vi "GetClusterElementByName(DBL).vi"(10 "ElementName":string[](array[string]), 11 "Cluster":variant) -> (2 "Found":bool, 3 "ValueOut":dbl)   [LabVIEW 2020, in "GetClusterElementByName.lvlib"]
uses:
  GetClusterElementByName.lvlib
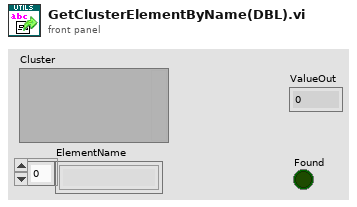
[diagram p1: front panel]
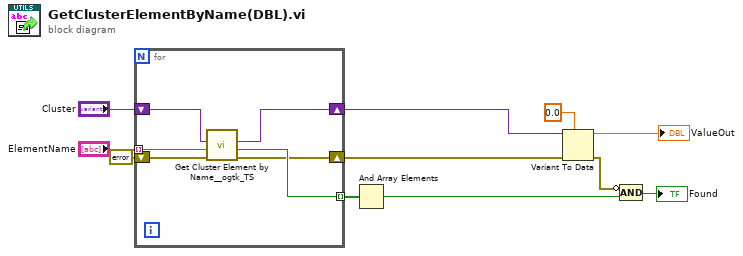
[diagram p0: block diagram]
diagram:
  n1 = for {
    tunnel: "ElementName" -> [w17] mode=indexing
    shift-right: [w16] -> w8
    shift-left: "Cluster" -> [w15]
    tunnel: [w14] -> w9 mode=indexing
    shift-right: [w13] -> w6
    shift-left: errorcluster {"status"=FALSE, "code"=0, "source"=""} ("error out") -> [w12]
    n2 = call "Get Cluster Element by Name__ogtk_TS.vi"("error in (no error)"=w12, "Element Name"=w17, "Cluster"=w15) -> ("error out"=w13:errorcluster, "found?"=w14:bool, "VElement"=w16:variant)  [unwired: 6 in]
  }
  n3 = And Array Elements(Boolean array=w9) -> (logical AND=w5:bool)
  n4 = Variant To Data(error in=w6, type=0.0, Variant=w8) -> (data=→"ValueOut":dbl, error out=w3:errorcluster)
  n5 = Compound Arithmetic op=AND(invert w3, w5) -> (→"Found":bool)
